vi "Update Configuration Command.vi"(8 "error in":errorcluster, 10 "Config JSON":string, 11 "CoreOOB_Rx in":refnum<class "CIFTemplateCoreOOB_Rx.lvclass">) -> (0 "error out":errorcluster, 3 "CoreOOB_Rx out":refnum<class "CIFTemplateCoreOOB_Rx.lvclass">)   [LabVIEW 2021, in "CIFTemplateCoreOOB_Rx.lvclass"]
uses:
  CIFTemplateCoreOOB_Rx.lvclass
  D:/dev/CIF-Core-LabVIEW/src/CIFUtilities/CifOutOfBand/CIFOutOfBand.lvclass
  CIFUtilities/CifOutOfBand/CIFOutOfBand.lvclass/CIFOutOfBand.ctl
  Typedef/OOB Core Commands.ctl
  Typedef/Template Payload.ctl
  CIFTemplateCoreOOB_Rx.lvclass/CIFTemplateCoreOOB_Rx.ctl
  CIFUtilities/CifOutOfBand/CIFOutOfBand.lvclass
  <vilib>/addons/_JKI.lib/Serialization/JSON/JKI JSON Serialization.lvlib
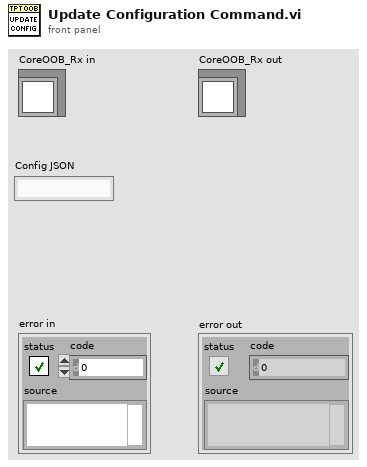
[diagram p1: front panel]
types:
  T1 = typedef "CIFTemplateCoreOOB_Rx.lvclass/OOB Core Commands.ctl" = enum8{"Start", "StartFTE", "Pause", "Stop", "Restart", "RestartFTE", "RefreshStats", "UpdateConfig"}
  T2 = typedef "CIFTemplateCoreOOB_Rx.lvclass/Template Payload.ctl" = cluster{"Config Data":variant, "FTE":u64}
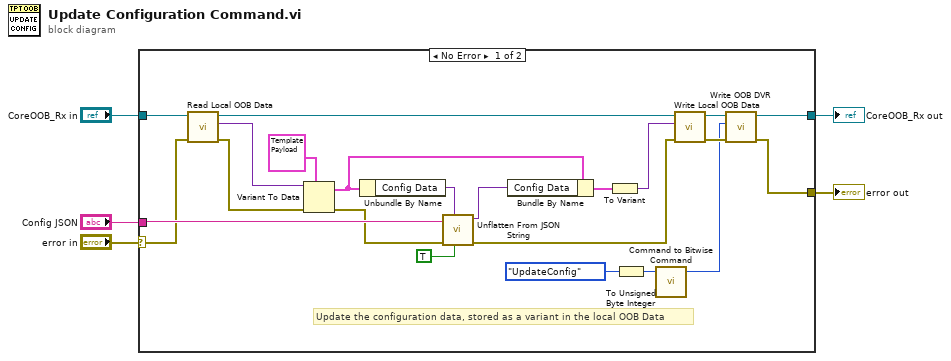
[diagram p0: block diagram]
diagram:
  n1 = case shown="No Error" "error in" {
    selector: "error in" -> [w19 w29]
    tunnel: [w26 w29] -> w4
    tunnel: "CoreOOB_Rx in" -> [w21 w28]
    tunnel: [w27 w28] -> w2
    tunnel: "Config JSON" -> [w25 _]
    frame No Error {
      # "Update the configuration data, stored as a variant in the local OOB Data"
      n2 = call "Read Local OOB Data.vi"("error in"=w19, "OOB in"=w21) -> ("error out"=w14:errorcluster, "Local OOB Data"=w18:variant, "OOB out"=w20:refnum<class "CIFTemplateCoreOOB_Rx.lvclass">)  [unwired: 7 in]
      n3 = Variant To Data(error in=w14, type=T2 {"Config Data"=variant, "FTE"=0} ("Template Payload"), Variant=w18) -> (data=w15:T2, error out=w13:errorcluster)
      n4 = Unbundle By Name(w15) -> ("Config Data"=w16:variant)
      n5 = call <vilib>:"Unflatten From JSON String.vi"("Nulls as Defaults (F)"=TRUE, "Type and Defaults"=w16, "error in (no error)"=w13, "JSON String"=w25) -> ("error out"=w24:errorcluster, "Variant"=w23:variant)  [unwired: 6 in]
      n6 = Bundle By Name(cluster=w15, "Config Data"=w23) -> (w8:T2)
      n7 = To Variant(anything=w8) -> (Variant=w7:variant)
      n8 = To Unsigned Byte Integer(number=OOB_Core_Commands."UpdateConfig" ("OOB Main Commands")) -> (unsigned 8bit integer=w10:u8)
      n9 = call "Command to Bitwise Command.vi"("OOB Command"=w10) -> ("bit command"=w6:u64)  [unwired: 3 in]
      n10 = call "Write Local OOB Data.vi"("error in"=w24, "Local OOB Data"=w7, "OOB in"=w20) -> ("error out"=w12:errorcluster, "OOB out"=w11:refnum<class "CIFTemplateCoreOOB_Rx.lvclass">)  [unwired: 7 in]
      n11 = call "Write OOB DVR.vi"("error in"=w12, "Commands (bitwise)"=w6, "OOB in"=w11) -> ("error out"=w26:errorcluster, "OOB out"=w27:refnum<class "CIFTemplateCoreOOB_Rx.lvclass">)  [unwired: 7 in]
    }
    frame Error {
    }
  }
  "error out" <- w4
  "CoreOOB_Rx out" <- w2
